vi "Control Icons.vi"(8 "Error In":errorcluster, 11 "VI In":refnum<vi>) -> (0 "Error Out":errorcluster, 2 "Control Icons":T1(array[cluster]), 3 "VI Out":refnum<vi>)   [LabVIEW 2018, in "Scripts.lvlib"]
uses:
  Scripts.lvlib
  <vilib>/Utility/traverseref.llb/TRef TravTarget.ctl
  <vilib>/Utility/traverseref.llb/VI Scripting - Traverse.lvlib
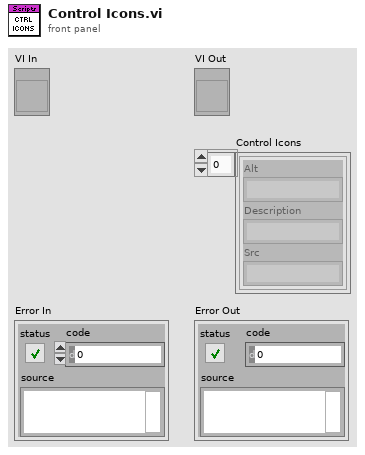
[diagram p1: front panel]
types:
  T1 = cluster{"Alt":string, "Description":string, "Src":string}[]
  T2 = typedef "TRef TravTarget.ctl" = enum16{"FP", "BD", "Other"}
  T3 = cluster{"String":string, "Paragraph Description":string, string}
  T4 = cluster{"String":string, "Paragraph Description":string, string}[]
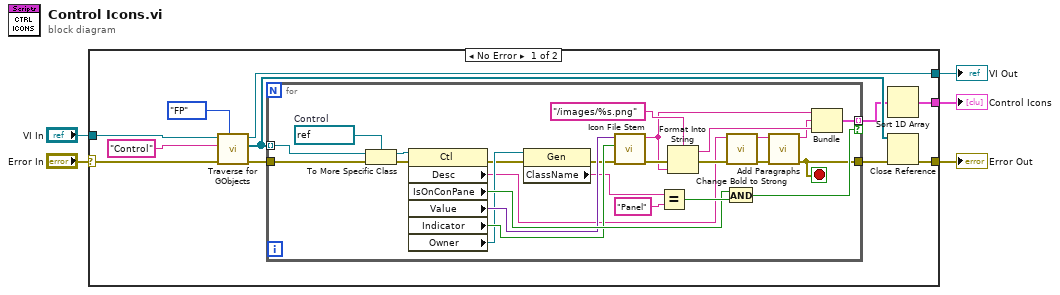
[diagram p0: block diagram]
diagram:
  n1 = case shown="No Error" "Error In" {
    selector: "Error In" -> [w12 w44]
    tunnel: [w10 w44] -> w5
    tunnel: "VI In" -> [w13 w43]
    tunnel: [w8 w43] -> w2
    tunnel: [w6 _] -> w1
    frame No Error {
      n2 = call <vilib>:"Traverse for GObjects.vi"("Traverse Target"=TRef_TravTarget."FP", "error in (no error)"=w12, "Class Name"="Control", "VI Refnum"=w13) -> ("error out"=w11:errorcluster, "References"=w9:refnum<vi>[], "dup VI Refnum"=w8:refnum<vi>)  [unwired: 4 in, 1 out]
      n3 = for {
        tunnel: w11 -> [w42]
        tunnel: [w19] -> w16
        tunnel: w9 -> [w27] mode=indexing
        tunnel: [w22] -> w7 mode=indexing if=w21
        stop <- w19 stop-if-true
        w37 = refnum<vi> refnum  # Control
        n4 = To More Specific Class(target class=w37, reference=w27, error in=w42) -> (specific class reference=w39:refnum<vi>, error out=w38:errorcluster)
        n5 = property class="Ctl"(reference=w39, error in=w38) -> (error out=w31:errorcluster, "Desc"=w25:string, "IsOnConPane"=w40:bool, "Value"=w34:variant, "Indicator"=w36:bool, "Owner"=w32:refnum<vi>)  [unwired: 1 out]
        n6 = property class="Gen"(reference=w32, error in=w31) -> (error out=w30:errorcluster, "ClassName"=w29:string)  [unwired: 1 out]
        n7 = call "Icon File Stem.vi"("Error In"=w30, "Indicator"=w36, "Value"=w34) -> ("Error Out"=w35:errorcluster, "String"=w23:string)  [unwired: 7 in]
        n8 = Equal?(x=w29, y="Panel") -> (x = y?=w41:bool)
        n9 = Format Into String(format string="/images/%s.png", error in=w35, w23) -> (resulting string=w24:string, error out=w26:errorcluster)  [unwired: 1 in]
        n10 = And(x=w40, y=w41) -> (x .and. y?=w21:bool)
        n11 = call "Change Bold to Strong.vi"("Error In"=w26, "Bold Description"=w25) -> ("Error Out"=w20:errorcluster, "Strong Description"=w18:string)  [unwired: 8 in]
        n12 = call "Add Paragraphs.vi"("Error In"=w20, "Multiple Newline Description"=w18) -> ("Error Out"=w19:errorcluster, "Paragraph Description"=w17:string)  [unwired: 8 in]
        n13 = Bundle("String"=w23, "Paragraph Description"=w17, w24) -> (w22:T3)  [unwired: 1 in]
      }
      n14 = Sort 1D Array(array=w7) -> (sorted array=w6:T4)
      n15 = Close Reference(reference=w9, error in (no error)=w16) -> (error out=w10:errorcluster)
    }
    frame Error {
    }
  }
  "Error Out" <- w5
  "VI Out" <- w2
  "Control Icons" <- w1
